vi "Decode.vi"(8 "Error In":errorcluster, 10 "Data":string, 11 "reference in":refnum<class "EncryptionDecorator.lvclass">) -> (0 "Error Out":errorcluster, 2 "Return(STRING)":string, 3 "reference in":refnum<class "EncryptionDecorator.lvclass">)   [LabVIEW 2020, in "EncryptionDecorator.lvclass"]
uses:
  EncryptionDecorator.lvclass
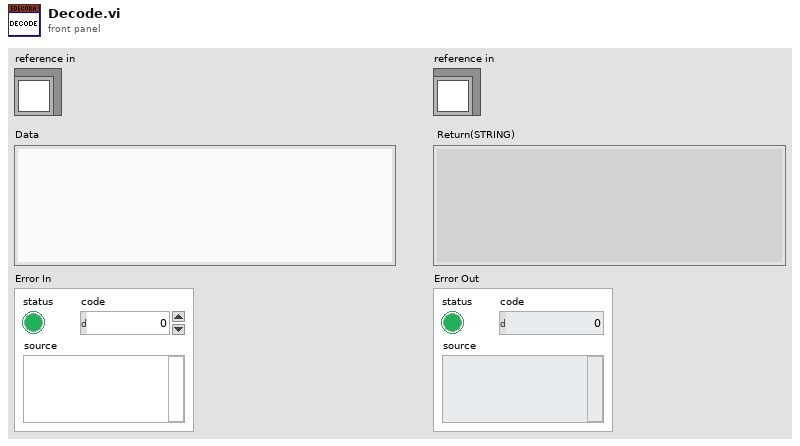
[diagram p1: front panel]
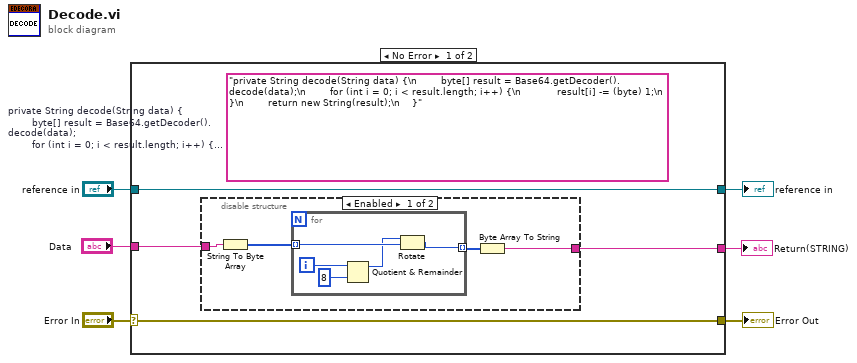
[diagram p0: block diagram]
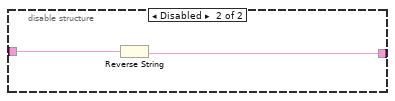
[diagram p2: hidden frame]
diagram:
  n1 = case shown="No Error" "Error In" {
    selector: "Error In" -> [w10 w23]
    tunnel: [w10 w23] -> w5
    tunnel: [w9 w22] -> w3
    tunnel: "reference in" -> [w9 w22]
    tunnel: "Data" -> [w8 _]
    tunnel: [w7 _] -> w1
    frame No Error {
      (unwired) "private String decode(String data) {\n        byte[] result = Base64.getDecoder().decode(data);\n        for (int i = 0; i < result.length; i++) {\n            result[i] -= (byte) 1;\n        }\n        return new String(result);\n    }"  # private String decode(String data) {         byte[] result = Base64.getDecoder().decode(data);         for (int i = 0; i < result.length; i++) {             result[i] -= (byte) 1;         }         return new String(result);     }
      n2 = disable-structure shown="Enabled" {
        disable-tunnel: w8 -> [w12 w21]
        disable-tunnel: [w11 w20] -> w7
        frame Enabled {
          n3 = String To Byte Array(string=w12) -> (unsigned byte array=w13:u8[])
          n4 = for {
            tunnel: w13 -> [w17] mode=indexing
            tunnel: [w16] -> w14 mode=indexing
            i -> [w19]
            n5 = Quotient & Remainder(x=w19, y=8) -> (x-y*floor(x/y)=w15:i32)  [unwired: 1 out]
            n6 = Rotate(1:w17, 2:w15) -> (0:w16:u8)
          }
          n7 = Byte Array To String(unsigned byte array=w14) -> (string=w11:string)
        }
        frame Disabled {
          n8 = Reverse String(1:w21) -> (0:w20:string)
        }
      }
    }
    frame Error {
    }
  }
  "Error Out" <- w5
  "reference in" <- w3
  "Return(STRING)" <- w1
